vi "SimpleRegister.vi"() -> ()   [LabVIEW 2021]
uses:
  <userlib>/SciSDK/SciSDK_Labview.lvlib
panel:
  out "Register C Value":u32
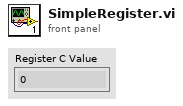
[diagram p1: front panel]
types:
  T1 = cluster{"Name":string, "Board Model":string, "Handle":u64}
  T2 = cluster{"Board Name":string, "Board Model":string, "SciSDK Handle":u64}
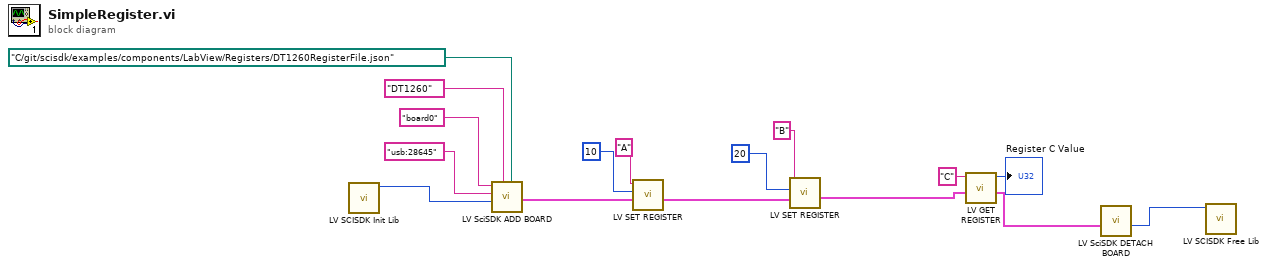
[diagram p0: block diagram]
diagram:
  n1 = call <userlib>:"LV SCISDK Init Lib.vi"() -> ("function return"=w16:u64)  [unwired: 11 in]
  n2 = call <userlib>:"LV SciSDK ADD BOARD.vi"("JsonFile"=path "C:/git/scisdk/examples/components/LabView/Registers/DT1260RegisterFile.json", "Board Model"="DT1260", "SciSDK Handle"=w16, "DevicePath"="usb:28645", "Name"="board0") -> ("Board Handle Out"=w8:T1)  [unwired: 4 in, 2 out]
  n3 = call <userlib>:"LV SET REGISTER.vi"("Board Handle In"=w8, "Value"=u32 10, "Name"="A") -> ("Board Handle Out"=w7:T1)  [unwired: 6 in, 2 out]
  n4 = call <userlib>:"LV SET REGISTER.vi"("Board Handle In"=w7, "Value"=u32 20, "Name"="B") -> ("Board Handle Out"=w5:T1)  [unwired: 6 in, 2 out]
  n5 = call <userlib>:"LV GET REGISTER.vi"("Board Handle In"=w5, "Register Name"="C") -> ("Board Handle Out"=w1:T2, "Register Value"=→"Register C Value":u32)  [unwired: 7 in, 1 out]
  n6 = call <userlib>:"LV SciSDK DETACH BOARD.vi"("Board Handle In"=w1) -> ("SciSDK Handle"=w2:u64)  [unwired: 9 in, 1 out]
  n7 = call <userlib>:"LV SCISDK Free Lib.vi"("handle"=w2) -> ()  [unwired: 9 in, 2 out]
